vi "Build Origin Map.vi"(8 "error in (no error)":errorcluster, 11 "Map Model in":refnum<class "Map Model.lvclass">) -> (0 "error out":errorcluster, 3 "Map Model out":refnum<class "Map Model.lvclass">)   [LabVIEW 2020, in "Map Model.lvlib" / "Map Model.lvclass"]
uses:
  Map Model.lvclass
  <vilib>/Utility/miscctls.llb/LVPoint32TypeDef.ctl
  Map Model.lvclass/Map Model.ctl
panel:
  # "NOTICE -- YOU MUST LEAVE THIS NOTICE IN PLACE.\n\nCopyright (c) 2017, LIANG LIU Shawn.Liu.cn@gmail.com\nAll rights reserved.\n\nRedistribution and use in source and binary forms, with or without modification, are permitted provided that the following conditions are met:\n-Redistributions of source code must retain the above copyright notice, this list of conditions and the following disclaimer.\n-Redistributions in binary form must reproduce the above copyright notice, this list of conditions and the following disclaimer in the documentation and/or other materials provided with the distribution.\n-Neither the name of the eLp nor the names of its contributors may be used to endorse or promote products derived from this software without specific prior written permission.\n\nTHIS SOFTWARE IS PROVIDED BY THE COPYRIGHT HOLDERS AND CONTRIBUTORS \"AS IS\" AND ANY EXPRESS OR IMPLIED WARRANTIES, INCLUDING, BUT NOT LIMITED TO, THE IMPLIED WARRANTIES OF MERCHANTABILITY AND FITNESS FOR A PARTICULAR PURPOSE ARE DISCLAIMED. IN NO EVENT SHALL THE COPYRIGHT HOLDER OR CONTRIBUTORS BE LIABLE FOR ANY DIRECT, INDIRECT, INCIDENTAL, SPECIAL, EXEMPLARY, OR CONSEQUENTIAL DAMAGES (INCLUDING, BUT NOT LIMITED TO, PROCUREMENT OF SUBSTITUTE GOODS OR SERVICES; LOSS OF USE, DATA, OR PROFITS; OR BUSINESS INTERRUPTION) HOWEVER CAUSED AND ON ANY THEORY OF LIABILITY, WHETHER IN CONTRACT, STRICT LIABILITY, OR TORT (INCLUDING NEGLIGENCE OR OTHERWISE) ARISING IN ANY WAY OUT OF THE USE OF THIS SOFTWARE, EVEN IF ADVISED OF THE POSSIBILITY OF SUCH DAMAGE."
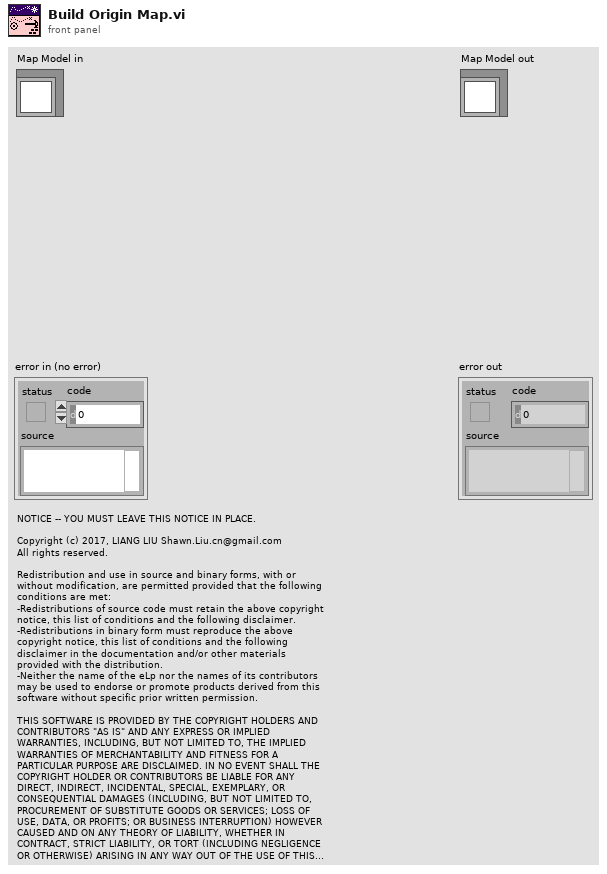
[diagram p1: front panel]
types:
  T1 = typedef "LVPoint32TypeDef.ctl" = cluster{"Horizontal":i32, "Vertical":i32}
  T2 = cluster{"Width":u16, "Style":enum32{"Solid", "Dash", "Dot", "DashDot", "DashDotDot"}}
  T3 = cluster{"Occupied Color":cluster{"Value":u8, "Color":u32}, "Free Color":cluster{"Value":u8, "Color":u32}, "Unknown Color":cluster{"Value":u8, "Color":u32}}
  T4 = typedef "LVPointTypeDef.ctl" = cluster{"Horizontal":i16, "Vertical":i16}
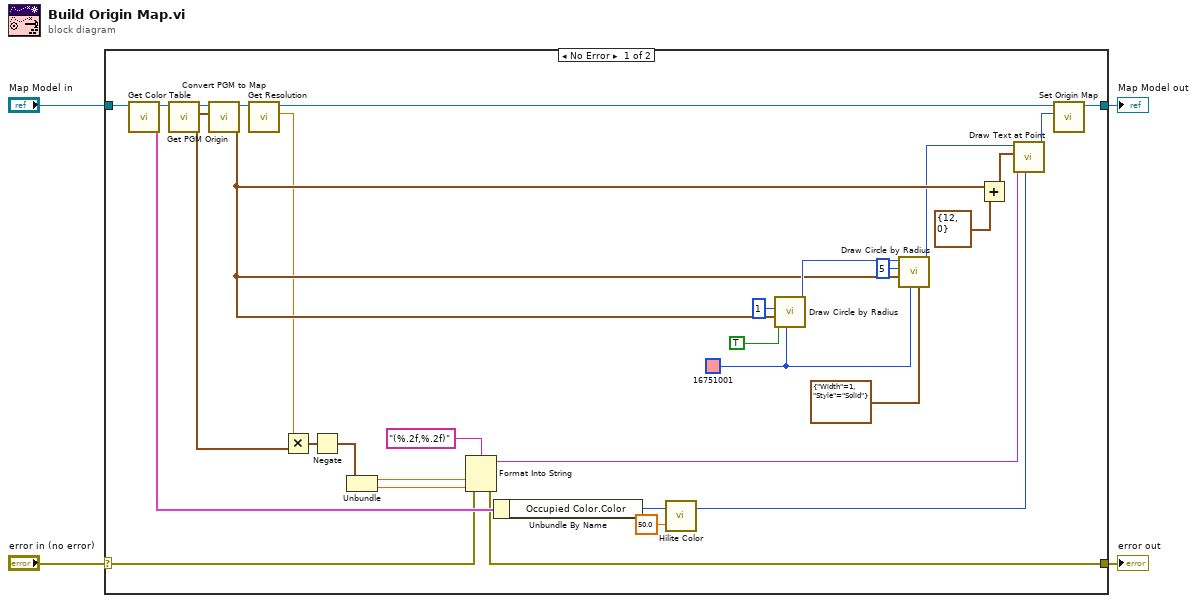
[diagram p0: block diagram]
diagram:
  n1 = case shown="No Error" "error in (no error)" {
    selector: "error in (no error)" -> [w6 w37]
    tunnel: [w21 w36] -> w4
    tunnel: "Map Model in" -> [w13 w36]
    tunnel: [w5 w37] -> w1
    frame No Error {
      w32 = u32 16751001 ("color(black)")
      n2 = call "Get Color Table.vi"("Map Model in"=w13) -> ("Color Table"=w12:T3, "Map Model out"=w14:refnum<class "Map Model.lvclass">)  [unwired: 9 in]
      n3 = call "Get PGM Origin.vi"("Map Model in"=w14) -> ("PGM Origin"=w22:cluster{"Horizontal":dbl, "Vertical":dbl}, "Map Model out"=w35:refnum<class "Map Model.lvclass">)  [unwired: 9 in]
      n4 = call "Convert PGM to Map.vi"("Position on PGM"=w22, "Map Model in"=w35) -> ("Position on Map"=w20:T4, "Map Model out"=w19:refnum<class "Map Model.lvclass">)  [unwired: 8 in]
      n5 = call "Get Resolution.vi"("Map Model in"=w19) -> ("Resolution"=w17:dbl, "Map Model out"=w8:refnum<class "Map Model.lvclass">)  [unwired: 9 in]
      n6 = Multiply(x=w17, y=w22) -> (x*y=w18:cluster{"Horizontal":dbl, "Vertical":dbl})
      n7 = Negate(x=w18) -> (-x=w16:cluster{"Horizontal":dbl, "Vertical":dbl})
      n8 = Unbundle(w16) -> ("Horizontal"=w28:dbl, "Vertical"=w27:dbl)
      n9 = Format Into String(format string="(%.2f,%.2f)", error in=w6, w28, w27) -> (resulting string=w11:string, error out=w5:errorcluster)  [unwired: 1 in]
      n10 = Unbundle By Name(w12) -> ("Occupied Color.Color"=w24:u32)
      n11 = call <vilib>:"Hilite Color.vi"("Percentage(30)"=50.0, "Color In"=w24) -> ("Hilite"=w25:u32)  [unwired: 1 out]
      n12 = call <vilib>:"Draw Circle by Radius.vi"("color(black)"=w32, "fill?(F)"=TRUE, "pixel center"=w20, "radius"=i16 1) -> ("new picture"=w34:picture)  [unwired: 7 in]
      n13 = call <vilib>:"Draw Circle by Radius.vi"("pen"=T2 {"Width"=1, "Style"=enum."Solid"}, "color(black)"=w32, "pixel center"=w20, "radius"=i16 5, "picture"=w34) -> ("new picture"=w15:picture)  [unwired: 6 in]
      n14 = Add(x=w20, y=T1 {"Horizontal"=12, "Vertical"=0}) -> (x+y=w10:T1)
      n15 = call <vilib>:"Draw Text at Point.vi"("text color(black)"=w25, "text"=w11, "origin"=w10, "picture"=w15) -> ("new picture"=w7:picture)  [unwired: 6 in, 1 out]
      n16 = call "Set Origin Map.vi"("Origin Map"=w7, "Map Model in"=w8) -> ("Map Model out"=w21:refnum<class "Map Model.lvclass">)  [unwired: 9 in]
    }
    frame Error {
    }
  }
  "error out" <- w1
  "Map Model out" <- w4
